vi "CRYSet Scope-FFT Front Panel.vi"(11 "Vi Ref in":refnum<vi> caption="Vi Ref") -> (3 "Vi Ref out":refnum<vi> caption="Vi Ref")   [LabVIEW 2013]
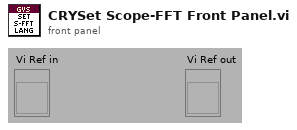
[diagram p1: front panel]
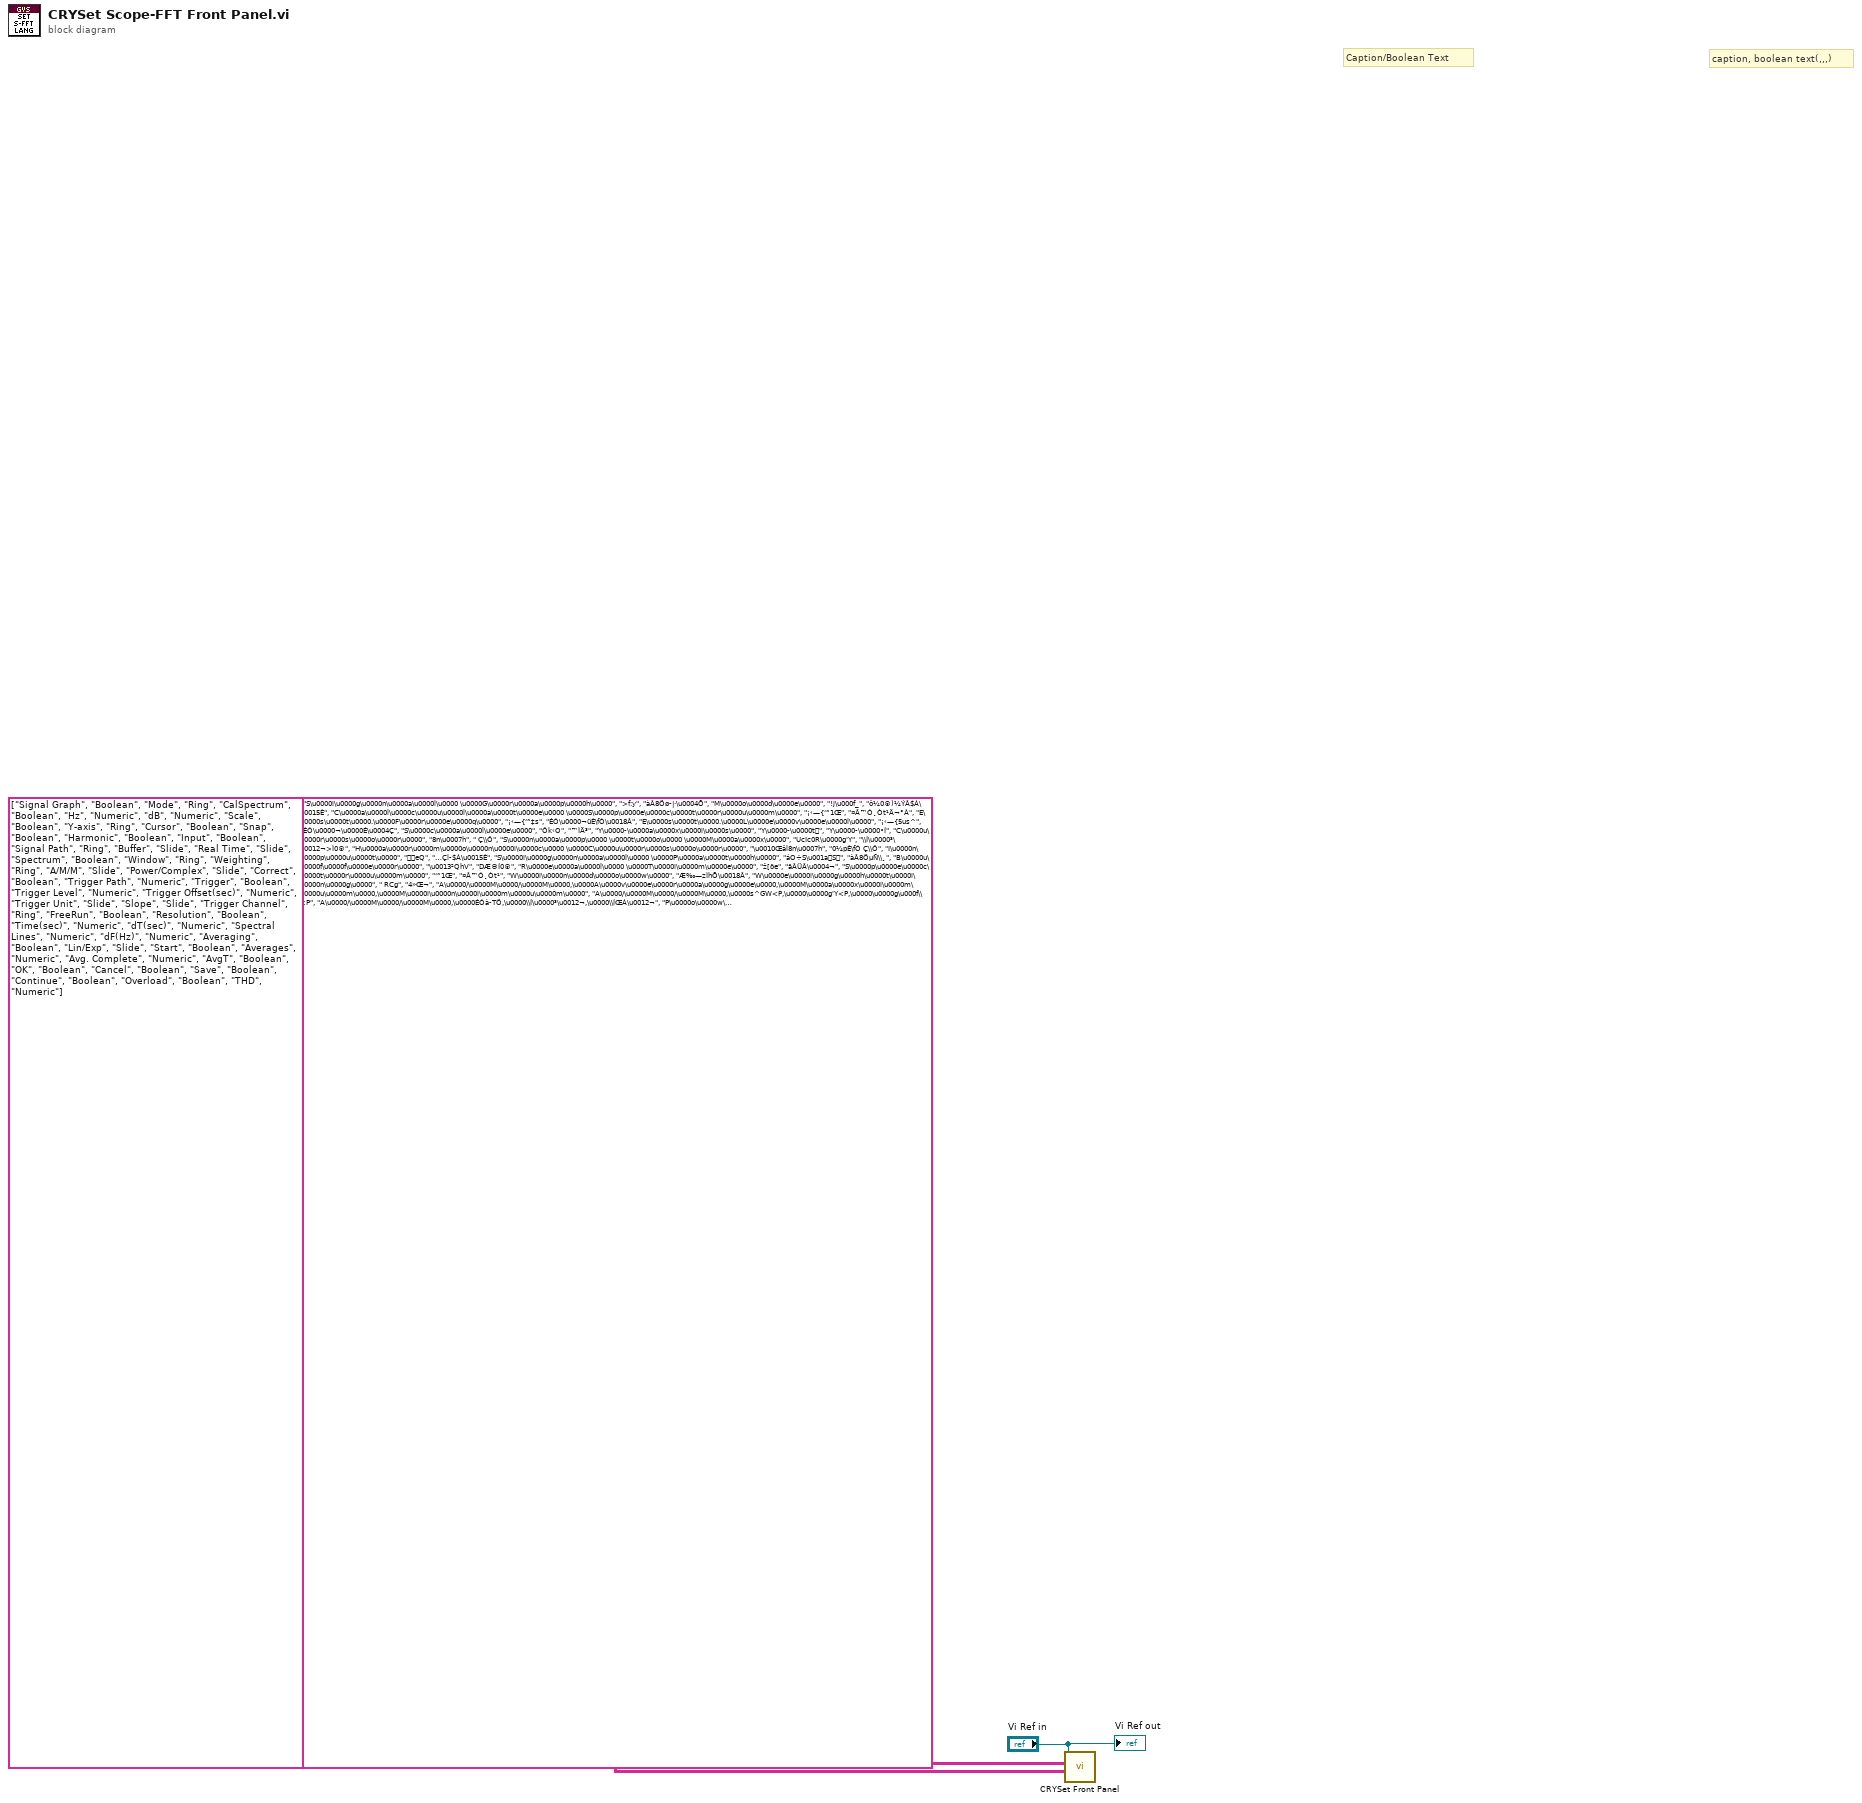
[diagram p0: block diagram]
diagram:
  # "caption, boolean text(,,,)"
  # "Caption/Boolean Text"
  n1 = call "CRYSet Front Panel.vi"("Caption(Boolean Text)"=string[][] [["S\u0000i\u0000g\u0000n\u0000a\u0000l\u0000 \u0000G\u0000r\u0000a\u0000p\u0000h\u0000", ">f:y", "àÂ8Öø­|·\u0004Õ"], ["M\u0000o\u0000d\u0000e\u0000", "!j\u000f_", "ô¼0®)¼ÝÂ$Á\u0015È"], ["C\u0000a\u0000l\u0000c\u0000u\u0000l\u0000a\u0000t\u0000e\u0000 \u0000S\u0000p\u0000e\u0000c\u0000t\u0000r\u0000u\u0000m\u0000", "¡‹—{‘˜1Œ", "¤Â™Ó¸Òt¹Ä¬°À"], ["E\u0000s\u0000t\u0000.\u0000F\u0000r\u0000e\u0000q\u0000", "¡‹—{‘˜‡s", "ÉÓ\u0000¬üÈ\fÓ\u0018Â"], ["E\u0000s\u0000t\u0000.\u0000L\u0000e\u0000v\u0000e\u0000l\u0000", "¡‹—{5us^", "ÉÓ\u0000¬\u0000É\u0004Ç"], ["S\u0000c\u0000a\u0000l\u0000e\u0000", "Ôk‹O", "™ÌÄ³"], ["Y\u0000-\u0000a\u0000x\u0000i\u0000s\u0000", "Y\u0000-\u0000t", "Y\u0000-\u0000•Í"], ["C\u0000u\u0000r\u0000s\u0000o\u0000r\u0000", "8n\u0007h", " Ç\\Ô"], ["S\u0000n\u0000a\u0000p\u0000 \u0000t\u0000o\u0000 \u0000M\u0000a\u0000x\u0000", "UcIc0R\u0000g'Y", "\\Í\u0000³\u0012¬>Ì0®"], ["H\u0000a\u0000r\u0000m\u0000o\u0000n\u0000i\u0000c\u0000 \u0000C\u0000u\u0000r\u0000s\u0000o\u0000r\u0000", "\u0010Œâl8n\u0007h", "0¼pÈ\fÓ Ç\\Ô"], ["I\u0000n\u0000p\u0000u\u0000t\u0000", "eQ", "…Çl­$Á\u0015È"], ["S\u0000i\u0000g\u0000n\u0000a\u0000l\u0000 \u0000P\u0000a\u0000t\u0000h\u0000", "áO÷S\u001aS", "àÂ8ÖµÑ\\¸"], ["B\u0000u\u0000f\u0000f\u0000e\u0000r\u0000", "\u0013²QhV", "DÆ©Í0®"], ["R\u0000e\u0000a\u0000l\u0000 \u0000T\u0000i\u0000m\u0000e\u0000", "ž[öe", "äÂÜÂ\u0004¬"], ["S\u0000p\u0000e\u0000c\u0000t\u0000r\u0000u\u0000m\u0000", "‘˜1Œ", "¤Â™Ó¸Òt¹"], ["W\u0000i\u0000n\u0000d\u0000o\u0000w\u0000", "Æ‰—z", "=ÌhÕ\u0018Â"], ["W\u0000e\u0000i\u0000g\u0000h\u0000t\u0000i\u0000n\u0000g\u0000", " RCg", "4»Œ¬"], ["A\u0000/\u0000M\u0000/\u0000M\u0000,\u0000A\u0000v\u0000e\u0000r\u0000a\u0000g\u0000e\u0000,\u0000M\u0000a\u0000x\u0000i\u0000m\u0000u\u0000m\u0000,\u0000M\u0000i\u0000n\u0000i\u0000m\u0000u\u0000m\u0000", "A\u0000/\u0000M\u0000/\u0000M\u0000,\u0000s^GW<P,\u0000\u0000g'Y<P,\u0000\u0000g\u000f\\<P", "A\u0000/\u0000M\u0000/\u0000M\u0000,\u0000ÉÓà­TÖ,\u0000\\Í\u0000³\u0012¬,\u0000\\ÍŒÁ\u0012¬"], ["P\u0000o\u0000w\u0000e\u0000r\u0000/\u0000C\u0000o\u0000m\u0000p\u0000l\u0000e\u0000x\u0000,\u0000P\u0000o\u0000w\u0000e\u0000r\u0000,\u0000C\u0000o\u0000m\u0000p\u0000l\u0000e\u0000x\u0000", "P\u0000o\u0000w\u0000e\u0000r\u0000/\u0000C\u0000o\u0000m\u0000p\u0000l\u0000e\u0000x\u0000,\u0000ŸR‡s,\u0000\rY\bT", "P\u0000o\u0000w\u0000e\u0000r\u0000/\u0000C\u0000o\u0000m\u0000p\u0000l\u0000e\u0000x\u0000,\u0000\u0004È%¸,\u0000õ¼ŒÁ\u0018Â"], ["A\u0000p\u0000p\u0000l\u0000y\u0000 \u0000C\u0000o\u0000r\u0000r\u0000e\u0000c\u0000t\u0000i\u0000o\u0000n\u0000", "”^(uîOck", "P­\u0000É\u0001È©Æ"], ["T\u0000r\u0000i\u0000g\u0000g\u0000e\u0000r\u0000 \u0000P\u0000a\u0000t\u0000h\u0000", "æÑS\u001aS", "¸Ò¬¹p¬µÑ\\¸"], ["T\u0000r\u0000i\u0000g\u0000g\u0000e\u0000r\u0000", "æ‰ÑS", "¸Ò¬¹p¬"], ["T\u0000r\u0000i\u0000g\u0000g\u0000e\u0000r\u0000 \u0000L\u0000e\u0000v\u0000e\u0000l\u0000", "æ‰ÑS5us^", "\u0000É\u0004Ç"], ["T\u0000r\u0000i\u0000g\u0000g\u0000e\u0000r\u0000 \u0000O\u0000f\u0000f\u0000s\u0000e\u0000t\u0000(\u0000s\u0000)\u0000", "æ‰ÑSOPûy(\u0000Òy)\u0000", "À¼\u0004Ç(\u0000\bÍ)\u0000"], ["T\u0000r\u0000i\u0000g\u0000g\u0000e\u0000r\u0000 \u0000U\u0000n\u0000i\u0000t\u0000,\u0000d\u0000B\u0000,\u0000V\u0000", "æ‰ÑSUSMO", "è²\u0004Ç,\u0000d\u0000B\u0000,\u0000V\u0000"], ["S\u0000l\u0000o\u0000p\u0000e\u0000", "œe‡s", "½¬¬À"], ["T\u0000r\u0000i\u0000g\u0000g\u0000e\u0000r\u0000 \u0000C\u0000h\u0000a\u0000n\u0000n\u0000e\u0000l\u0000", "æÑS\u001aS", "µÑ\\¸"], ["F\u0000r\u0000e\u0000e\u0000 \u0000R\u0000u\u0000n\u0000,\u0000T\u0000r\u0000i\u0000g\u0000g\u0000e\u0000r\u0000e\u0000d\u0000", "ê1uÐL,\u0000æÑS", "Ç \u0000Ù³,\u0000¸Ò¬¹p¬"], ["R\u0000e\u0000s\u0000o\u0000l\u0000u\u0000t\u0000i\u0000o\u0000n\u0000", "\u0006R¨s", "„½tÕ¥²"], ["T\u0000i\u0000m\u0000e\u0000(\u0000s\u0000e\u0000c\u0000)\u0000", "öeô•(\u0000Òy)\u0000", "ÜÂ\u0004¬(\u0000\bÍ)\u0000"], ["d\u0000T\u0000(\u0000s\u0000e\u0000c\u0000)\u0000", "d\u0000T\u0000(\u0000s\u0000e\u0000c\u0000)\u0000", "d\u0000T\u0000(\u0000s\u0000e\u0000c\u0000)\u0000"], ["S\u0000p\u0000e\u0000c\u0000t\u0000r\u0000a\u0000l\u0000 \u0000L\u0000i\u0000n\u0000e\u0000s\u0000", "‘˜1Œ¿~", "¤Â™Ó¸Òt¹ Á"], ["d\u0000F\u0000(\u0000H\u0000z\u0000)\u0000", "d\u0000F\u0000(\u0000H\u0000z\u0000)\u0000", "d\u0000F\u0000(\u0000H\u0000z\u0000)\u0000"], ["A\u0000v\u0000e\u0000r\u0000a\u0000g\u0000i\u0000n\u0000g\u0000", "s^GW", "ÉÓà­TÖ"], ["L\u0000i\u0000n\u0000/\u0000E\u0000x\u0000p\u0000,\u0000L\u0000i\u0000n\u0000e\u0000a\u0000r\u0000,\u0000E\u0000x\u0000p\u0000o\u0000n\u0000e\u0000n\u0000t\u0000i\u0000a\u0000l\u0000", "¿~'`/\u0000\u0007cpe,\u0000¿~'`,\u0000\u0007cpe", " Á\u0015Ö/\u0000ÀÉ\u0018Â,\u0000 Á\u0015Ö,\u0000ÀÉ\u0018Â"], ["S\u0000t\u0000a\u0000r\u0000t\u0000,\u0000S\u0000t\u0000o\u0000p\u0000", "\u0000_ËY,\u0000\\Pbk", "ÜÂ \u0000‘Ç,\u0000\u0015È \u0000ÀÉ"], ["A\u0000v\u0000e\u0000r\u0000a\u0000g\u0000e\u0000s\u0000", "s^GW", "ÉÓà­\u001c¬\u0018Â"], ["A\u0000v\u0000g\u0000.\u0000 \u0000C\u0000o\u0000m\u0000p\u0000l\u0000e\u0000t\u0000e\u0000", ";`s^GWpe", "ÉÓà­\\Õ \u0000\u001c¬\u0018Â"], ["A\u0000v\u0000e\u0000r\u0000a\u0000g\u0000i\u0000n\u0000g\u0000", "s^GW.\u0000.\u0000.\u0000", "ÉÓà­.\u0000.\u0000.\u0000"], ["O\u0000K\u0000", "nx¤‹", "UÖxÇ"], ["C\u0000a\u0000n\u0000c\u0000e\u0000l\u0000", "ÖSˆm", "èÍŒÁ"], ["S\u0000a\u0000v\u0000e\u0000 \u0000t\u0000o\u0000 \u0000 \u0000C\u0000u\u0000r\u0000v\u0000e\u0000L\u0000i\u0000b\u0000", "ÝOX[0Ròf¿~“^", "á¬ Á\u001cÁà¬ÐÅ \u0000ô¼\u0000­"], ["C\u0000o\u0000n\u0000t\u0000i\u0000n\u0000u\u0000e\u0000", "ç~ \u0000í~", "Ä¬ \u0000Á"], ["O\u0000V\u0000E\u0000R\u0000L\u0000O\u0000A\u0000D\u0000", "Ç \u0000}", "\\ÕÄ¬\u0018±hÎ"], ["T\u0000H\u0000D\u0000", ";`\u0010Œâl1Y\u001fw", "T\u0000H\u0000D\u0000"]], "Control ID and Type(Label Name, Type)"=string[][] [["Signal Graph", "Boolean"], ["Mode", "Ring"], ["CalSpectrum", "Boolean"], ["Hz", "Numeric"], ["dB", "Numeric"], ["Scale", "Boolean"], ["Y-axis", "Ring"], ["Cursor", "Boolean"], ["Snap", "Boolean"], ["Harmonic", "Boolean"], ["Input", "Boolean"], ["Signal Path", "Ring"], ["Buffer", "Slide"], ["Real Time", "Slide"], ["Spectrum", "Boolean"], ["Window", "Ring"], ["Weighting", "Ring"], ["A/M/M", "Slide"], ["Power/Complex", "Slide"], ["Correct", "Boolean"], ["Trigger Path", "Numeric"], ["Trigger", "Boolean"], ["Trigger Level", "Numeric"], ["Trigger Offset(sec)", "Numeric"], ["Trigger Unit", "Slide"], ["Slope", "Slide"], ["Trigger Channel", "Ring"], ["FreeRun", "Boolean"], ["Resolution", "Boolean"], ["Time(sec)", "Numeric"], ["dT(sec)", "Numeric"], ["Spectral Lines", "Numeric"], ["dF(Hz)", "Numeric"], ["Averaging", "Boolean"], ["Lin/Exp", "Slide"], ["Start", "Boolean"], ["Averages", "Numeric"], ["Avg. Complete", "Numeric"], ["AvgT", "Boolean"], ["OK", "Boolean"], ["Cancel", "Boolean"], ["Save", "Boolean"], ["Continue", "Boolean"], ["Overload", "Boolean"], ["THD", "Numeric"]], "Vi Ref"="Vi Ref in") -> ()  [unwired: 9 in]
  "Vi Ref out" <- "Vi Ref in"
